vi "LB_Open.vi"(8 "error in (no error)":errorcluster caption="错误输入（无错误）", 11 "LB_COM_IN":refnum<visa-resource-name>="COM4") -> (0 "error out":errorcluster caption="错误输出", 2 "OK":bool, 3 "LB_COM_OUT":refnum<visa-resource-name>)   [LabVIEW 2015, in "LBAnalyser.lvlib"]
uses:
  LBAnalyser.lvlib
  <vilib>/Instr/_visa.llb/VISA Configure Serial Port (Instr).vi
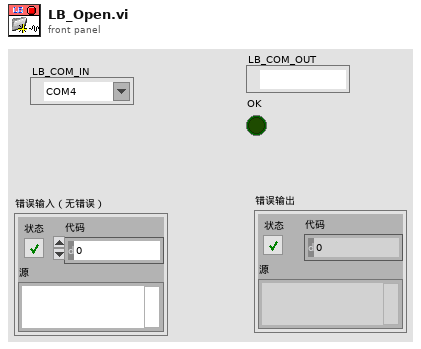
[diagram p1: front panel]
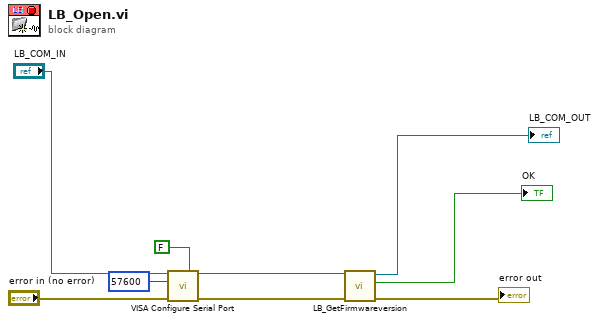
[diagram p0: block diagram]
diagram:
  n1 = call-poly "VISA Configure Serial Port"("VISA resource name"="LB_COM_IN", "Enable Termination\nChar (T)"=FALSE ("Enable Termination\nChar (T)"), "baud rate (9600)"=u32 57600, "error in (no error)"="error in (no error)") -> ("VISA resource name out"=w4:refnum<visa-resource-name>, "error out"=w5:errorcluster)  [unwired: 10 in]
  n2 = call "LB_GetFirmwareversion.vi"("error in (no error)"=w5, "LB_COM_IN"=w4) -> ("error out"=→"error out":errorcluster, "OK"=→"OK":bool, "LB_COM_OUT"=→"LB_COM_OUT":refnum<visa-resource-name>)  [unwired: 7 in]
